vi "InputUpdate.vi"() -> ()   [LabVIEW 2016]
uses:
  <vilib>/Rock Robotics/WPI/Utilities/WPI_GetSetVariantRefNum.vi
  Globals/InputValues.vi
  <vilib>/Rock Robotics/Network Tables/NT Write Boolean Array.vi
  <vilib>/Rock Robotics/Network Tables/NT Write Numeric Array.vi
  Globals/Constantes.vi
panel:
  out "OutputJoystick Y 2":dbl
  out "OutputJoystick X 2":dbl
  out "Triggers Combined Value":dbl
  in  "Use Triggers":bool
  out "OutputJoystick Y":dbl
  out "OutputJoystick X":dbl
  out "Joystick X":dbl
  out "Joystick Y":dbl
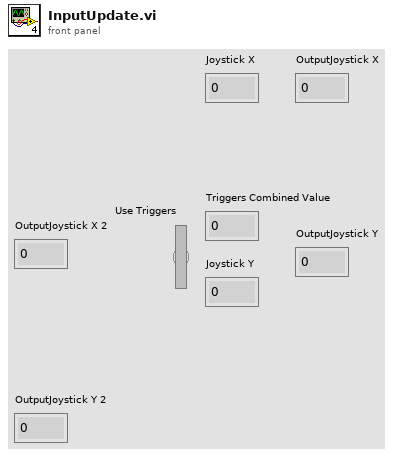
[diagram p1: front panel]
types:
  T1 = typedef "WPI_JoystickDevRef.ctl" = cluster{"Device":T2}
  T2 = typedef "WPI_JoystickDeviceEnum.ctl" = enum16{"USB 0", "USB 1", "USB 2", "USB 3", "USB 4", "USB 5"}
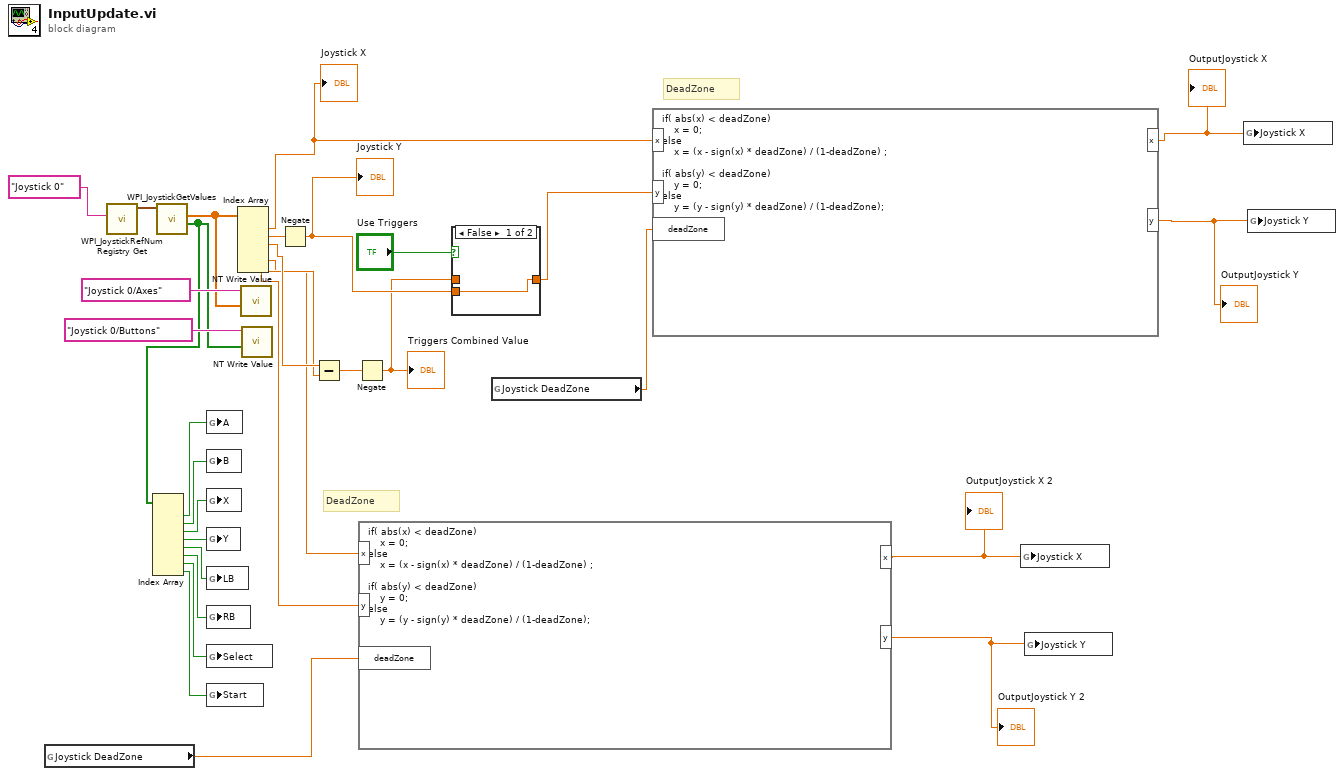
[diagram p0: block diagram]
diagram:
  # "DeadZone"
  # "DeadZone"
  n1 = global read "Constantes.vi" "Joystick DeadZone"() -> (w3:dbl)
  n2 = call <vilib>:"WPI_JoystickRefNum Registry Get.vi"("refnum name"="Joystick 0") -> ("JoystickDevRef"=w30:T1)  [unwired: 1 in, 9 out]
  n3 = call <vilib>:"WPI_JoystickGetValues.vi"("JoystickDevRef"=w30) -> ("Buttons"=w14:bool[], "Axes"=w27:dbl[])  [unwired: 6 in, 3 out]
  n4 = Index Array(array=w14) -> (element #1=w13:bool, element #2=w12:bool, element #3=w11:bool, element #4=w10:bool, element #5=w9:bool, element #6=w8:bool, element #7=w7:bool, element #8=w6:bool)  [unwired: 8 in]
  n5 = global write "InputValues.vi" "A"(w13) -> ()
  n6 = global write "InputValues.vi" "B"(w12) -> ()
  n7 = global write "InputValues.vi" "X"(w11) -> ()
  n8 = global write "InputValues.vi" "Y"(w10) -> ()
  n9 = global write "InputValues.vi" "LB"(w9) -> ()
  n10 = global write "InputValues.vi" "RB"(w8) -> ()
  n11 = global write "InputValues.vi" "Select"(w7) -> ()
  n12 = global write "InputValues.vi" "Start"(w6) -> ()
  n13 = Index Array(array=w27) -> (element #1=w25:dbl, element #2=w21:dbl, element #3=w19:dbl, element #4=w15:dbl, element #5=w5:dbl, element #6=w4:dbl)  [unwired: 6 in]
  "Joystick X" <- w25
  n14 = call-poly <vilib>:"NT Write Value.vi"("Numeric Array"=w27, "Name"="Joystick 0/Axes") -> ()  [unwired: 9 in, 1 out]
  n15 = call-poly <vilib>:"NT Write Value.vi"("Boolean Array"=w14, "Name"="Joystick 0/Buttons") -> ()  [unwired: 9 in, 1 out]
  n16 = Negate(x=w21) -> (-x=w17:dbl)
  "Joystick Y" <- w17
  n17 = Subtract(x=w19, y=w15) -> (x-y=w20:dbl)
  n18 = Negate(x=w20) -> (-x=w16:dbl)
  "Triggers Combined Value" <- w16
  n19 = formula code="if( abs(x) < deadZone)\n    x = 0;\nelse\n    x = (x - sign(x) * deadZone) / (1-deadZone) ;\n\nif( abs(y) < deadZone)\n    y = 0;\nelse\n    y = (y - sign(y) * deadZone) / (1-deadZone);"("y"=w4, "x"=w5, "deadZone"=w3) -> ("x"=w2:dbl, "y"=w1:dbl)
  "OutputJoystick X 2" <- w2
  "OutputJoystick Y 2" <- w1
  n20 = case shown="False" "Use Triggers" {
    tunnel: [w32 w33] -> w23
    tunnel: w17 -> [w32 _]
    tunnel: w16 -> [_ w33]
    frame False {
    }
    frame True {
    }
  }
  n21 = global read "Constantes.vi" "Joystick DeadZone"() -> (w26:dbl)
  n22 = formula code="if( abs(x) < deadZone)\n    x = 0;\nelse\n    x = (x - sign(x) * deadZone) / (1-deadZone) ;\n\nif( abs(y) < deadZone)\n    y = 0;\nelse\n    y = (y - sign(y) * deadZone) / (1-deadZone);"("y"=w23, "x"=w25, "deadZone"=w26) -> ("x"=w24:dbl, "y"=w18:dbl)
  "OutputJoystick X" <- w24
  "OutputJoystick Y" <- w18
  n23 = global write "InputValues.vi" "Joystick X"(w2) -> ()
  n24 = global write "InputValues.vi" "Joystick Y"(w1) -> ()
  n25 = global write "InputValues.vi" "Joystick X"(w24) -> ()
  n26 = global write "InputValues.vi" "Joystick Y"(w18) -> ()
